vi "OpenSubpanelHandler.vi"(8 "error in (no error)":errorcluster, 10 "GUID":string, 11 "SMO.UI.MAUI in":refnum<class "SMO.UI.MAUI.lvclass">) -> (0 "error out":errorcluster, 3 "SMO.UI.MAUI out":refnum<class "SMO.UI.MAUI.lvclass">)   [LabVIEW 2020, in "SMO.UI.MAUI.lvclass"]
uses:
  SMO.UI.MAUI.lvclass
  SMO.UI.MAUI.lvclass/SMO.UI.MAUI.ctl
  <vilib>/Levylab/SMO.UI.Embedded/SMO.UI.Embedded.lvclass
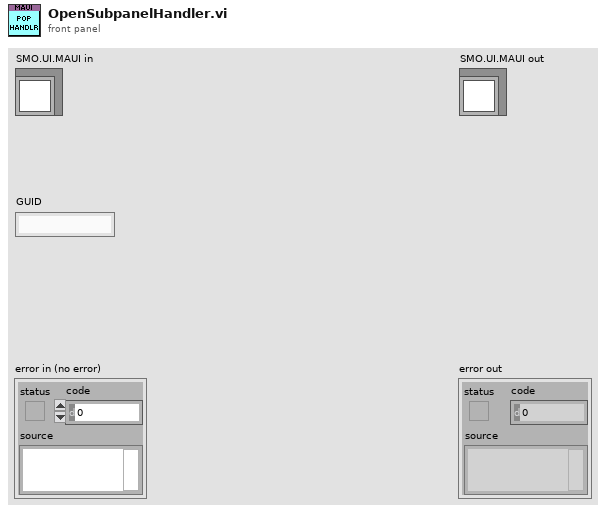
[diagram p1: front panel]
types:
  T1 = typedef "SMO.UI.MAUI.lvclass/PanelData.ctl" = cluster{"SubPanel":refnum<vi>, "Ring":refnum<vi>, "Active":i32}
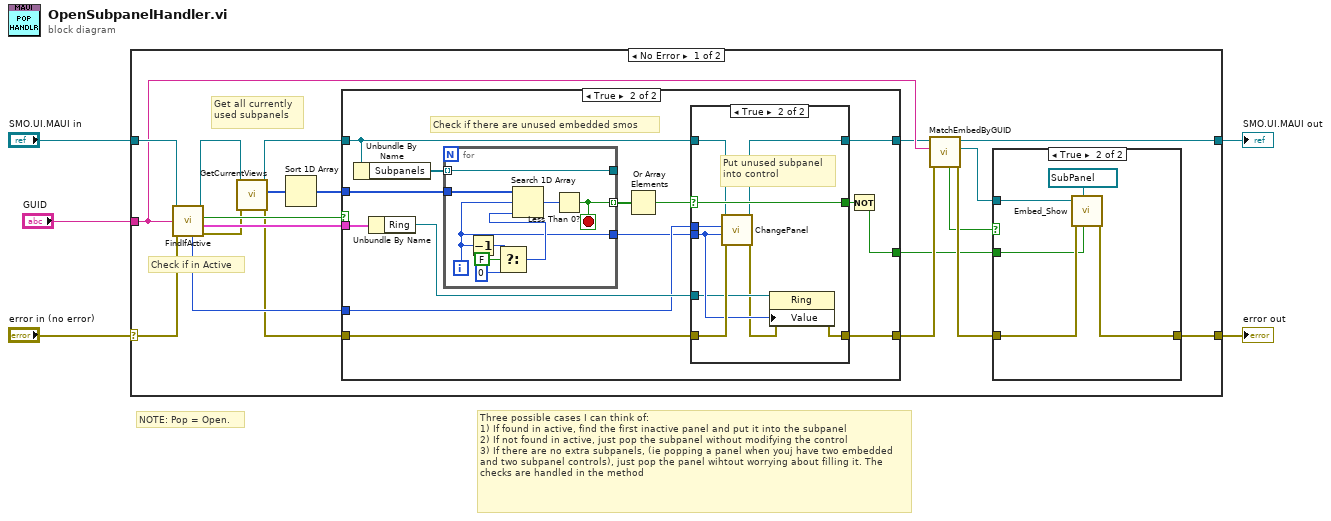
[diagram p0: block diagram]
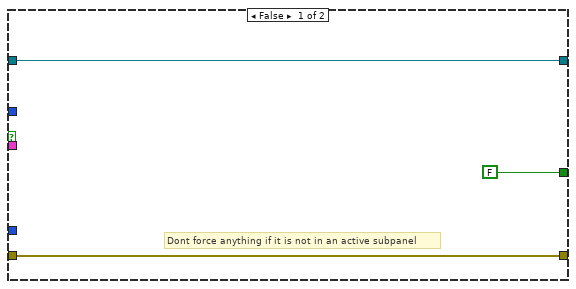
[diagram p3: hidden frame]
diagram:
  # "NOTE: Pop = Open."
  # "Three possible cases I can think of:\n1) If found in active, find the first inactive panel and put it into the subpanel\n2) If not found in active, just pop the subpanel without modifying the control\n3) If there are no extra subpanels, (ie popping a panel when youj have two embedded and two subpanel controls), just pop the panel wihtout worrying about filling it. The checks are handled in the method"
  n1 = case shown="No Error" "error in (no error)" {
    selector: "error in (no error)" -> [w24 w71]
    tunnel: [w9 w71] -> w4
    tunnel: [w11 w70] -> w2
    tunnel: "SMO.UI.MAUI in" -> [w25 w70]
    tunnel: "GUID" -> [w13 _]
    frame No Error {
      # "Get all currently used subpanels"
      # "Check if in Active"
      n2 = call "FindIfActive.vi"("error in (no error)"=w24, "GUID"=w13, "SMO.UI.MAUI in"=w25) -> ("error out"=w15:errorcluster, "Panel"=w19:T1, "Found?"=w20:bool, "SMO.UI.MAUI out"=w23:refnum<class "SMO.UI.MAUI.lvclass">, "Panel Index"=w17:i32)  [unwired: 4 in]
      n3 = call "GetCurrentViews.vi"("error in (no error)"=w15, "SMO.UI.MAUI in"=w23) -> ("error out"=w16:errorcluster, "Current Views"=w22:i32[], "SMO.UI.MAUI out"=w21:refnum<class "SMO.UI.MAUI.lvclass">)  [unwired: 7 in]
      n4 = Sort 1D Array(array=w22) -> (sorted array=w18:i32[])
      n5 = case shown="True" w20 {
        tunnel: w21 -> [w34 w47]
        tunnel: [w34 w48] -> w12
        tunnel: w19 -> [_ w42]
        tunnel: w18 -> [_ w45]
        tunnel: w17 -> [_ w40]
        tunnel: w16 -> [w33 w37]
        tunnel: [w33 w36] -> w14
        tunnel: [FALSE w35] -> w6
        frame False {
          # "Dont force anything if it is not in an active subpanel"
        }
        frame True {
          # "Check if there are unused embedded smos"
          n6 = Unbundle By Name(w47) -> ("Subpanels"=w46:refnum<class "SMO.UI.Embedded.lvclass">[])
          n7 = Unbundle By Name(w42) -> ("Ring"=w41:refnum<vi>)
          n8 = for {
            tunnel: w46 -> [w55] mode=indexing
            tunnel: w45 -> [w57]
            tunnel: [w54] -> w44 mode=indexing
            tunnel: [w49] -> w39
            tunnel: [w55] -> _
            i -> [w49]
            stop <- w54 stop-if-true
            n9 = Decrement(x=w49) -> (x-1=w53:i32)
            n10 = Select(t=w53, s=FALSE, f=0) -> (s? t:f=w50:i32)
            n11 = Search 1D Array(1D array=w57, element=w49, start index (0)=w50) -> (index of element=w56:i32)
            n12 = Less Than 0?(x=w56) -> (x < 0?=w54:bool)
          }
          n13 = Or Array Elements(Boolean array=w44) -> (logical OR=w43:bool)
          n14 = case shown="True" w43 {
            selector: w43 -> [w59 w69]
            tunnel: w47 -> [w60 w67]
            tunnel: [w60 w68] -> w48
            tunnel: w41 -> [_ w62]
            tunnel: w40 -> [_ w66]
            tunnel: w39 -> [_ w64]
            tunnel: [w59 w69] -> w38
            tunnel: w37 -> [w58 w65]
            tunnel: [w58 w63] -> w36
            frame False {
            }
            frame True {
              # "Put unused subpanel\ninto control"
              n15 = call "ChangePanel.vi"("error in (no error)"=w65, "New Active Index"=w64, "Panel Index"=w66, "MAUI in"=w67) -> ("error out"=w61:errorcluster, "MAUI out"=w68:refnum<class "SMO.UI.MAUI.lvclass">)  [unwired: 6 in]
              n16 = property class="Ring"(reference=w62, error in=w61, "Value"=w64) -> (error out=w63:errorcluster)  [unwired: 1 out]
            }
          }
          n17 = Not(x=w38) -> (.not. x?=w35:bool)
        }
      }
      n18 = call "MatchEmbedByGUID.vi"("error in (no error)"=w14, "GUID"=w13, "SMO.UI.MAUI in"=w12) -> ("error out"=w10:errorcluster, "Value"=w7:refnum<class "SMO.UI.Embedded.lvclass">, "SMO.UI.MAUI out"=w11:refnum<class "SMO.UI.MAUI.lvclass">, "Found?"=w8:bool)  [unwired: 4 in, 1 out]
      n19 = case shown="True" w8 {
        tunnel: w10 -> [w26 w28]
        tunnel: [w26 w29] -> w9
        tunnel: w7 -> [_ w31]
        tunnel: w6 -> [_ w27]
        frame False {
          # "If you dont find subpanel,\nDont stick it into reference."
        }
        frame True {
          n20 = call <vilib>:"Embed_Show.vi"("Force?"=w27, "Sub Panel"=refnum<vi> refnum, "error in (no error)"=w28, "EmbeddedSMO in"=w31) -> ("error out"=w29:errorcluster)  [unwired: 6 in, 1 out]
        }
      }
    }
    frame Error {
    }
  }
  "error out" <- w4
  "SMO.UI.MAUI out" <- w2
